vi "Analyze Replace Pattern.vi"(0 "Replace Pattern":string) -> (1 "Replace Constants":string[](array[string]), 2 "Replace Variable Indexes":i32[](array[numeric]))   [LabVIEW 2020]
doc: "Decomposes a Replace Pattern.\n\n<B>Replace Pattern</B> - The pattern to decompose.\n<B>Replace Constants</B> - The constant strings, split by this $n indexes.\n<B>Replace Variable Indexes</B> - The index in the Search Pattern parenthesized list to insert.\n\nThe two arrays are intended to be \"interleaved,\" with <B>Replace Constants</B> contributing to the first and last elements of the merged string. There will always be n+1 elements in <B>Replace Constants</B> where n is the number of elements in <B>Replace Variable Indexes</B>."
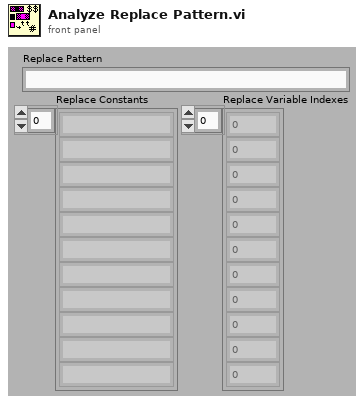
[diagram p1: front panel]
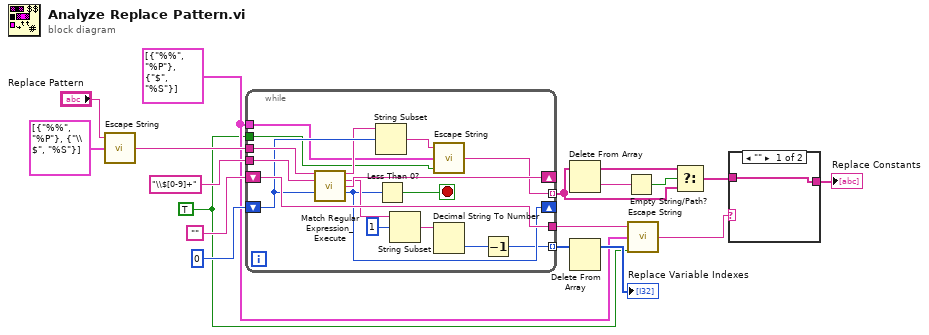
[diagram p0: block diagram]
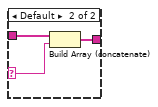
[diagram p2: hidden frame]
diagram:
  w8 = cluster{"String":string, "Escape":string}[] [{"String"="%%", "Escape"="%P"}, {"String"="$", "Escape"="%S"}] ("Escapes")
  w7 = TRUE ("replace all? (F)")
  n1 = call <vilib>:"Escape String.vi"("Escapes"=cluster{"String":string, "Escape":string}[] [{"String"="%%", "Escape"="%P"}, {"String"="\\$", "Escape"="%S"}], "String in"="Replace Pattern") -> ("String out"=w11:string)  [unwired: 1 out]
  n2 = while {
    tunnel: w11 -> [w35]
    tunnel: "\\$[0-9]+" ("regular expression") -> [w34]
    shift-right: [w25] -> _
    shift-left: 0 ("whole match offset") -> [w27]
    shift-right: [w33] -> _
    shift-left: "" -> [w32]
    tunnel: [w24] -> w3 mode=indexing
    tunnel: [w32] -> w9
    tunnel: [w19] -> w16 mode=indexing
    tunnel: w7 -> [w23]
    tunnel: w8 -> [w22]
    stop <- w31 stop-if-true
    n3 = call <vilib>:"Match Regular Expression_Execute.vi"("input string"=w35, "regular expression"=w34, "offset (0)"=w27) -> ("before match"=w26:string, "whole match"=w28:string, "after match"=w33:string, "whole match offset"=w25:i32)  [unwired: 3 in, 6 out]
    n4 = String Subset(string=w26, offset (0)=w27) -> (substring=w21:string)  [unwired: 1 out]
    n5 = Less Than 0?(x=w25) -> (x < 0?=w31:bool)
    n6 = String Subset(string=w28, offset (0)=1) -> (substring=w29:string)  [unwired: 1 out]
    n7 = call <vilib>:"Escape String.vi"("Remove Escapes? (False)"=w23, "Escapes"=w22, "String in"=w21) -> ("String out"=w24:string)
    n8 = Decimal String To Number(string=w29) -> (number=w20:i32)  [unwired: 3 out]
    n9 = Decrement(x=w20) -> (x-1=w19:i32)
  }
  n10 = Delete From Array(array=w3) -> (deleted portion=w6:string, array with subset deleted=w4:string[])  [unwired: 2 in]
  n11 = Delete From Array(array=w16) -> (array with subset deleted=→"Replace Variable Indexes":i32[])  [unwired: 2 in, 1 out]
  n12 = Empty String/Path?(string/path=w6) -> (empty?=w5:bool)
  n13 = call <vilib>:"Escape String.vi"("Remove Escapes? (False)"=w7, "Escapes"=w8, "String in"=w9) -> ("String out"=w2:string)
  n14 = Select(t=w4, s=w5, f=w3) -> (s? t:f=w1:string[])
  n15 = case shown="\"\"" w2 {
    selector: w2 -> [_ w37]
    tunnel: [w36 w39] -> w17
    tunnel: w1 -> [w36 w38]
    frame "" {
    }
    frame Default {
      n16 = Build Array (concatenate)(w38, w37) -> (w39:string[])
    }
  }
  "Replace Constants" <- w17
